vi "get_fiducials.vi"(10 "Calibration task":T2) -> (2 "Fiducial points":T1)   [LabVIEW 2014]
uses:
  asap/labview/testing/calibration_task.ctl
  <vilib>/Analysis/Matrix/Datatypes/RealMatrix.ctl
  asap/labview/initialization/globals.vi
  <vilib>/Analysis/Matrix/NI_Matrix.lvlib
panel:
  in  "Maxon hack":bool
  # "Return the fiducial points for a particular light calibration procedure."
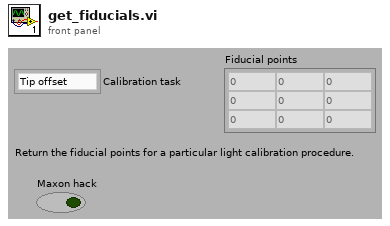
[diagram p1: front panel]
types:
  T1 = typedef "NI_Matrix.lvlib/RealMatrix.ctl" = dbl[][]
  T2 = typedef "calibration_task.ctl" = enum16{"Tip offset", "RCM offset", "Tip lights", "Handle lights"}
  T3 = enum16{"ASAP/Trigger", "ASAP/Finder", "ASAP/Micron", "ASAP/Micron 2", "Micron 6DOF"}
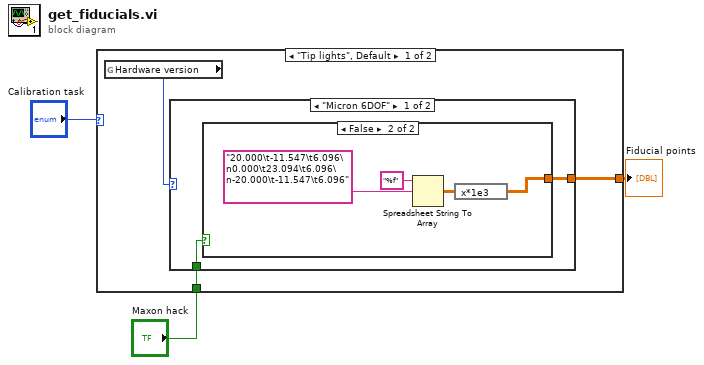
[diagram p0: block diagram]
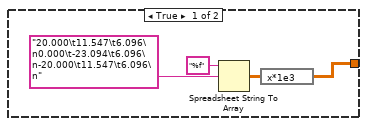
[diagram p2: hidden frame]
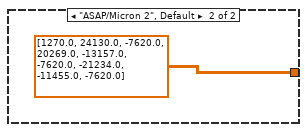
[diagram p3: hidden frame]
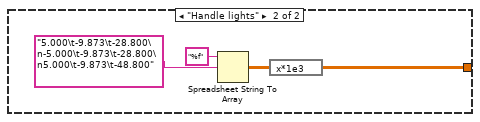
[diagram p4: hidden frame]
diagram:
  n1 = case shown="\"Tip lights\", Default" "Calibration task" {
    tunnel: [w5 w18] -> w2
    tunnel: "Maxon hack" -> [w4 _]
    frame "Tip lights", Default {
      n2 = global read "globals.vi" "Hardware version"() -> (w6:T3)
      n3 = case shown="\"Micron 6DOF\"" w6 {
        tunnel: [w8 T1 [[1270.0, 24130.0, -7620.0], [20269.0, -13157.0, -7620.0], [-21234.0, -11455.0, -7620.0]] ("Reference points")] -> w5
        tunnel: w4 -> [w7 _]
        frame "Micron 6DOF" {
          n4 = case shown="False" w7 {
            tunnel: [w9 w13] -> w8
            frame True {
              n5 = Spreadsheet String To Array(format string="%f", spreadsheet string="20.000\t11.547\t6.096\n0.000\t-23.094\t6.096\n-20.000\t11.547\t6.096\n") -> (array=w12:dbl[][])  [unwired: 2 in]
              n6 = expression code="x*1e3"(w12) -> (w9:dbl[][])
            }
            frame False {
              n7 = Spreadsheet String To Array(format string="%f", spreadsheet string="20.000\t-11.547\t6.096\n0.000\t23.094\t6.096\n-20.000\t-11.547\t6.096") -> (array=w16:dbl[][])  [unwired: 2 in]
              n8 = expression code="x*1e3"(w16) -> (w13:dbl[][])
            }
          }
        }
        frame "ASAP/Micron 2", Default {
        }
      }
    }
    frame "Handle lights" {
      n9 = Spreadsheet String To Array(format string="%f", spreadsheet string="5.000\t-9.873\t-28.800\n-5.000\t-9.873\t-28.800\n5.000\t-9.873\t-48.800") -> (array=w21:dbl[][])  [unwired: 2 in]
      n10 = expression code="x*1e3"(w21) -> (w18:dbl[][])
    }
  }
  "Fiducial points" <- w2
